vi "uploadExample.vi"() -> ()   [LabVIEW 2016, in "GDrive.lvlib"]
doc: "Example that demonstrates how to upload a file from local machine to Google Drive"
uses:
  VIs/GDrive.lvlib
panel:
  in  "Name of File on Drive":string
  in  "Local Path":path
  in  "Path to Secret Client JSON":path
  # "Provide the path to secret client JSON, the path to the file the user wants \nto upload, and the desired name of the file once it's on the drive. \nThis information is\nsufficient to upload the file specified by the local path."
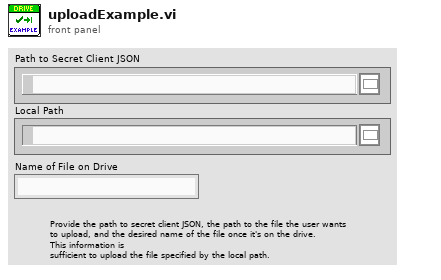
[diagram p1: front panel]
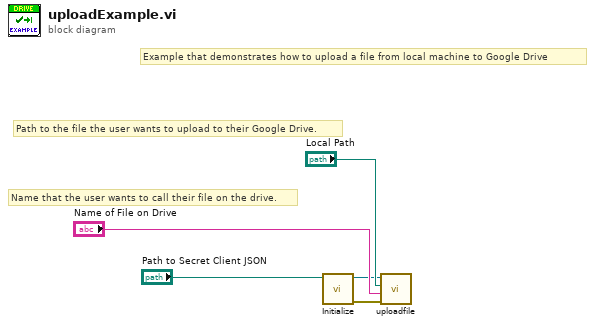
[diagram p0: block diagram]
diagram:
  # "Name that the user wants to call their file on the drive."
  # "Path to the file the user wants to upload to their Google Drive."
  # "Example that demonstrates how to upload a file from local machine to Google Drive"
  n1 = call "Initialize.vi"("Path to Secret Client JSON"="Path to Secret Client JSON") -> ("error out"=w4:errorcluster, "Google Drive Service Ref"=w1:refnum<k24>)  [unwired: 9 in]
  n2 = call "uploadfile.vi"("error in (no error)"=w4, "File Name on Drive"="Name of File on Drive", "Local Path"="Local Path", "Google Drive Service Ref"=w1) -> ()  [unwired: 6 in, 1 out]
